vi "(SubVI)Serial_COM port Check1.vi"(7 "Auto Detect?":bool, 8 "error in (no error)":errorcluster caption="에러 입력(에러 없음)", 9 "ID to Exclude":u8 format="%.0x", 10 "ID to Find":u8 format="%.0x", 11 "VISA resource name":refnum<visa-resource-name>) -> (0 "error out":errorcluster caption="에러 출력", 1 "IC Type":T2, 2 "BD Version":T1 {"BD FW Version" format="%08x"}, 3 "VISA resource name out":refnum<visa-resource-name>, 4 "I2C Slave ID":cluster{string, u8}[](array[cluster]), 5 "BD Info Str":string, 6 "Default I2C Slave ID":u8)   [LabVIEW 2020]
uses:
  Libraries/Haptic IC Class/Haptic IC/Controls/(Ctrl)IC Type.ctl
  <vilib>/Instr/_visa.llb/VISA Find Search Mode.ctl
  Controls/(Ctrl)Serial_FGV Function.ctl
  5283ad07-9809-4087-83e9-a87157ce31b4.vi
  <vilib>/Comparison/Equal/Equal Functor/Equal Functor.lvclass
  Libraries/Haptic IC Class/Haptic IC/Haptic IC.lvclass
panel:
  # "(SubVI)Serial_COM port Check.vi By hspark\n\nDescription : VISA Serial 연결 후 Board Information 명령어로 Board HW Version, FW Version, Chip ID 리스트 등을 얻는 VI\n\nInput : \n1. VISA resource name : 사용자가 선택한 COM port\n2. Auto Detect? : True 입력 시 VISA resource name 입력을 무시하고 PC에 연결되어 있는 모든 COM port에 대해 Checking 진행\n                        순차적으로 진행 중 Board를 찾으면 중지함\n3. ID to Find : 9786 등과 같이 Chip ID 확인이 불가능한 IC의 경우, 찾으려는 ID를 입력받아서 ID List에 있는 경우 해당 ID가 선택되게 함\n\nOutput : \n1. VISA resource name out : 연결된 COM port 출력\n2. BD FW Version : U32로 된 Board의 FW Version\n3. BD HW Version : 프로토콜에 명시된 Board의 HW Version (모델 추가 시 열거형 타입 정의 업데이트)\n4. I2C Slave ID : Board로부터 수신받은 I2C Slave ID 목록. 링 컨트롤 업데이트를 위한 클러스터 배열 출력.\n5. Default I2C Slave ID : Chip ID가 있는 첫번째 Slave ID. 모든 Slave가 Chip ID가 없는 경우 첫번째 Slave ID\n\nLabVIEW Version : 2020 SP1 이상\n\nNote :\n\nUpdate : 2021.12.20"
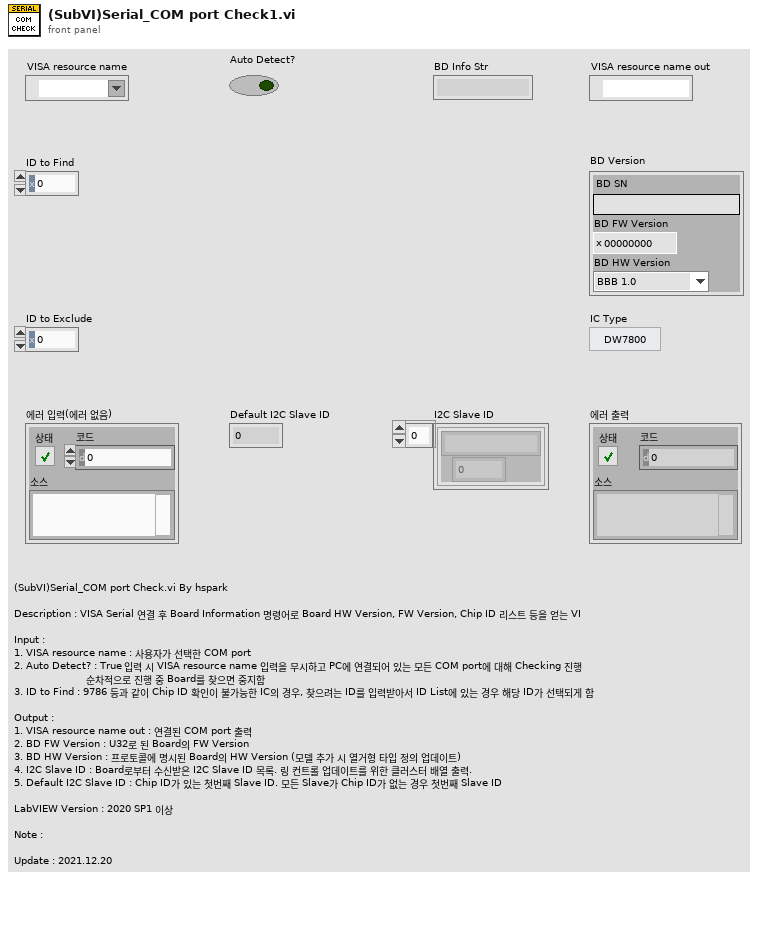
[diagram p1: front panel]
types:
  T1 = cluster{"BD SN":string, "BD FW Version":u32, "BD HW Version":enum8{"BBB 1.0", "BBB 1.1", "WBB 1.0", "reserved", "RedNoah3"}}
  T2 = typedef "Haptic IC.lvclass/(Ctrl)IC Type.ctl" = enum8{"DW7800", "DW7802", "DW7912", "DW7914"}
  T3 = typedef "(Ctrl)Serial_FGV Function.ctl" = enum16{"Initialize", "Read", "Read All", "Write", "Flush Buffer", "Get Ref.", "Close"}
  T4 = typedef "VISA Find Search Mode.ctl" = u32
  T5 = enum8{"BBB 1.0", "BBB 1.1", "WBB 1.0", "reserved", "RedNoah3"}
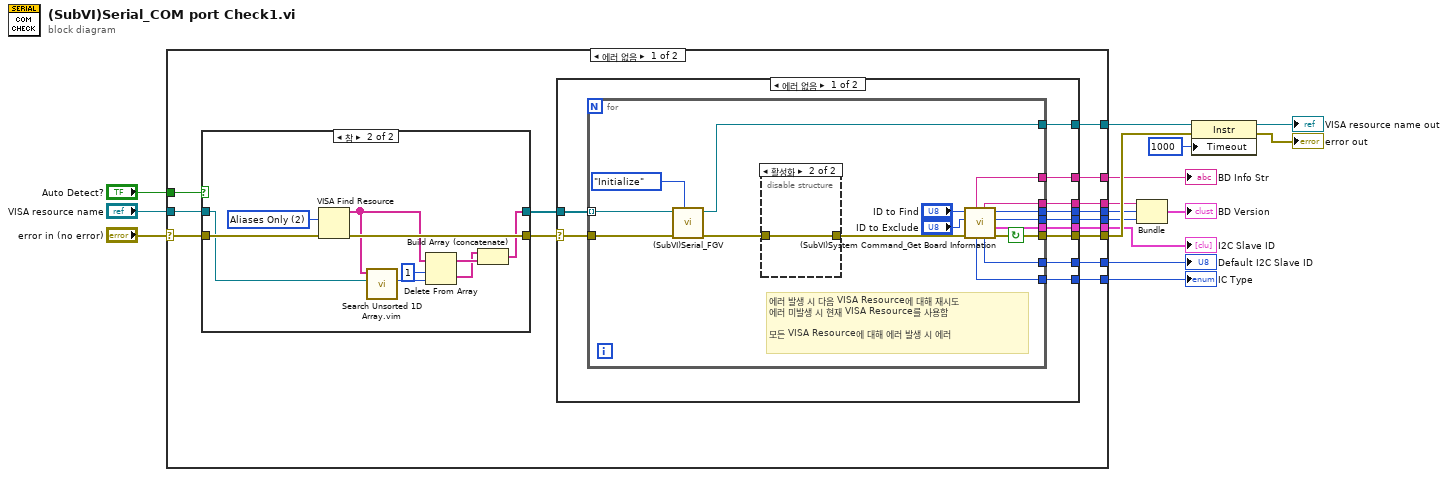
[diagram p0: block diagram]
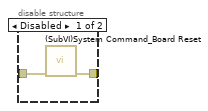
[diagram p2: hidden frame]
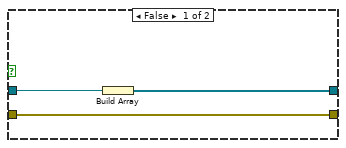
[diagram p4: hidden frame]
diagram:
  n1 = case shown="에러 없음" "error in (no error)" {
    selector: "error in (no error)" -> [w29 w76]
    tunnel: [w27 w76] -> w15
    tunnel: [w26 _] -> w3
    tunnel: [w25 _] -> w4
    tunnel: "Auto Detect?" -> [w24 _]
    tunnel: "VISA resource name" -> [w23 w75]
    tunnel: [w22 _] -> w12
    tunnel: [w21 _] -> w11
    tunnel: [w20 w75] -> w8
    tunnel: [w19 _] -> w10
    tunnel: [w18 _] -> w5
    tunnel: [w17 _] -> w1
    frame No Error {
      n2 = case shown="참" w24 {
        tunnel: w23 -> [w64 w71]
        tunnel: [w63 w65] -> w30
        tunnel: w29 -> [w62 w73]
        tunnel: [w62 w72] -> w28
        frame False {
          n3 = Build Array(w64) -> (w63:refnum<visa-resource-name>[])
        }
        frame True {
          w74 = T4 2 items=["Canonical Names Only"=0, "Aliases Only"=2, "Include Matching Aliases"=3, "Include All Aliases"=4] ("Search Mode")
          n4 = VISA Find Resource(8:w73, 10:w74) -> (0:w72:errorcluster, 3:w70:string[])  [unwired: 1 in, 1 out]
          n5 = call "Search Unsorted 1D Array.vim"("element"=w71, "unsorted 1D array"=w70) -> ("index of element"=w69:i32)  [unwired: 9 in]
          n6 = Delete From Array(array=w70, length=1 ("길이"), index=w69) -> (deleted portion=w66:string[], array with subset deleted=w67:string[])
          n7 = Build Array (concatenate)(w66, w67) -> (w65:string[])
        }
      }
      n8 = case shown="에러 없음" w28 {
        selector: w28 -> [w40 w61]
        tunnel: w30 -> [w41 _]
        tunnel: [w39 w61] -> w27
        tunnel: [w38 _] -> w26
        tunnel: [w37 _] -> w25
        tunnel: [w36 _] -> w22
        tunnel: [w35 _] -> w21
        tunnel: [w34 _] -> w20
        tunnel: [w33 _] -> w19
        tunnel: [w32 _] -> w18
        tunnel: [w31 _] -> w17
        frame No Error {
          n9 = for {
            tunnel: [w55] -> w37
            tunnel: [w54] -> w38
            tunnel: w41 -> [w53] mode=indexing
            tunnel: [w52] -> w39
            tunnel: w40 -> [w51]
            tunnel: [w50] -> w36
            tunnel: [w49] -> w35
            tunnel: [w48] -> w34
            tunnel: [w43] -> w33
            tunnel: [w44] -> w32
            tunnel: [w42] -> w31
            stop <- w52 continue-if-true
            # "에러 발생 시 다음 VISA Resource에 대해 재시도\n에러 미발생 시 현재 VISA Resource를 사용함 \n\n모든 VISA Resource에 대해 에러 발생 시 에러"
            n10 = call "(SubVI)Serial_FGV.vi"("Function"=(Ctrl)Serial_FGV_Function."Initialize", "error in (no error)"=w51, "VISA resource name"=w53) -> ("error out"=w56:errorcluster, "VISA resource name out"=w48:refnum<visa-resource-name>)  [unwired: 6 in, 1 out]
            n11 = disable-structure shown="활성화" {
              disable-tunnel: w56 -> [w59 w60]
              disable-tunnel: [w58 w60] -> w45
              frame Disabled {
                n12 = call "(SubVI)System Command_Board Reset.vi"("error in (no error)"=w59) -> ("error out"=w58:errorcluster)  [unwired: 9 in, 1 out]
              }
              frame Enabled {
              }
            }
            n13 = call "(SubVI)System Command_Get Board Information.vi"("error in (no error)"=w45, "ID to Exclude"="ID to Exclude", "ID to Find"="ID to Find") -> ("error out"=w52:errorcluster, "I2C Slave ID"=w50:cluster{string, u8}[], "BD HW Version"=w54:T5, "BD FW Version"=w55:u32, "Default I2C Slave ID"=w49:u8, "BD SN"=w42:string, "IC Type"=w44:T2, "BD Info Str"=w43:string)  [unwired: 1 in]
          }
        }
        frame Error {
        }
      }
    }
    frame Error {
    }
  }
  "I2C Slave ID" <- w12
  "Default I2C Slave ID" <- w11
  "BD Info Str" <- w10
  "IC Type" <- w5
  n14 = Bundle("BD SN"=w1, "BD FW Version"=w4, "BD HW Version"=w3) -> (→"BD Version":T1)  [unwired: 1 in]
  n15 = property class="Instr"(reference=w8, error in=w15, "Timeout"=u32 1000 ("General Settings:Timeout Value")) -> (reference out=→"VISA resource name out":refnum<visa-resource-name>, error out=→"error out":errorcluster)
